vi "Make Accel JSON.vi"(9 "Force":bool, 10 "Previous":T1={"type"="AI", "device"="", "name"="", "data"={"<init"=FALSE, "<range"=0.0, ">x"=0.0, ">y"=0.0, ">z"=0.0}}, 11 "New":T1={"type"="AI", "device"="", "name"="", "data"={"<init"=FALSE, "<range"=0.0, ">x"=0.0, ">y"=0.0, ">z"=0.0}}) -> (3 "delta JSON":string)   [LabVIEW 2019]
uses:
  Accel proto.ctl
  Accel Data proto.ctl
panel:
  out "Complete JSON":string
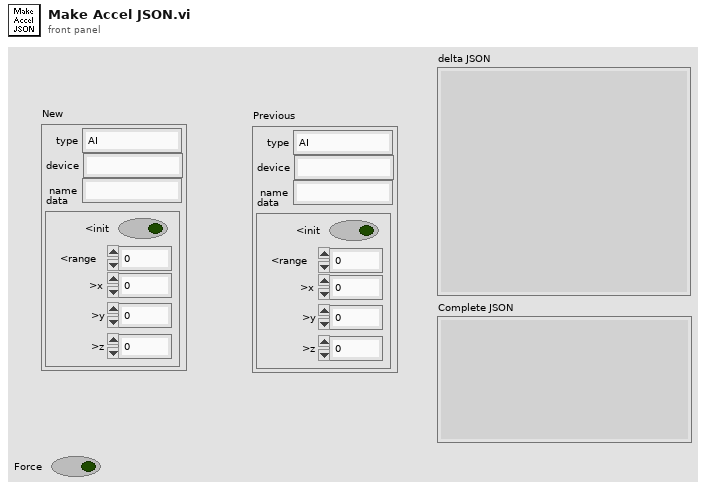
[diagram p1: front panel]
types:
  T1 = typedef "Accel proto.ctl" = cluster{"type":string, "device":string, "name":string, "data":T2}
  T2 = typedef "Accel Data proto.ctl" = cluster{"<init":bool, "<range":dbl, ">x":dbl, ">y":dbl, ">z":dbl}
  T3 = cluster{"type":bool, "device":bool, "name":bool, "data":cluster{"<init":bool, "<range":bool, ">x":bool, ">y":bool, ">z":bool}}
  T4 = cluster{"<init":bool, "<range":bool, ">x":bool, ">y":bool, ">z":bool}
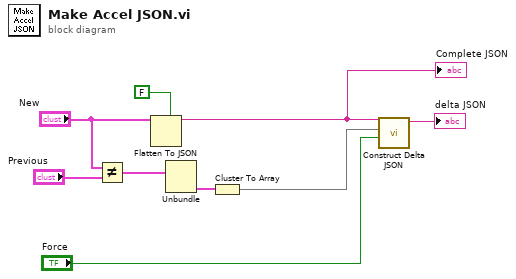
[diagram p0: block diagram]
diagram:
  n1 = Not Equal?(x="New", y="Previous") -> (x != y?=w6:T3)
  n2 = Flatten To JSON(enable LabVIEW extensions? (T)=FALSE, anything="New") -> (JSON string=w5:string)  [unwired: 1 in, 1 out]
  "Complete JSON" <- w5
  n3 = Unbundle(w6) -> ("data"=w2:T4)  [unwired: 3 out]
  n4 = Cluster To Array(cluster=w2) -> (array=w1:bool[])
  n5 = call "Construct Delta JSON.vi"("Force"="Force", "Checked Items"=w1, "JSON string"=w5) -> ("Delta JSON"=→"delta JSON":string)  [unwired: 8 in]
